vi "Configure Histogram Trigger Source.vi"(8 "error in (no error)":errorcluster {"code" format="%.0x"}, 9 "Histogram Trigger Source (1: Software)":i32(ring)=1 items=["External", "Software", "Immediate", "Pin 1", "Pin 2", "Pin 3"], 10 "Channel Name (1)":string="1", 11 "VISA resource name":refnum<visa-resource-name>) -> (0 "error out":errorcluster {"code" format="%.0x"}, 3 "VISA resource name out":refnum<visa-resource-name>)   [LabVIEW 2010, in "Agilent N6700 Series.lvlib"]
doc: "Configures the trigger source of the histogram function. When the power supply receives a trigger signal on the source you specify, it runs the histogram.\n\n<b>Note:</b>\n\n(1) The VI only applies to models N6781A and N6782A that have the Data Logger function installed.\n\n(2) The histogram function only applies to the N6705B DC Power Analyzer."
uses:
  Agilent N6700 Series.lvlib
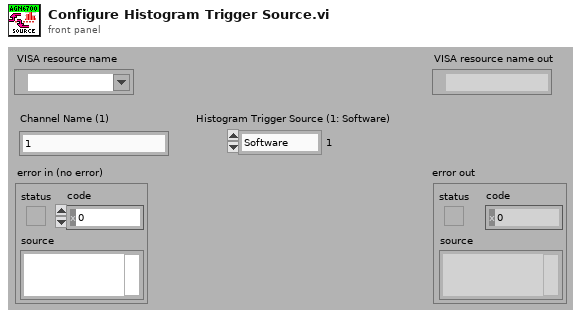
[diagram p1: front panel]
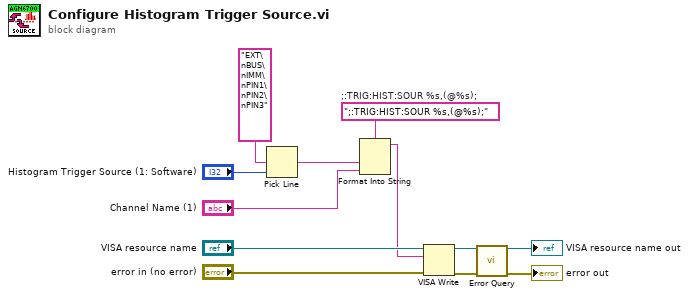
[diagram p0: block diagram]
diagram:
  w12 = ";:TRIG:HIST:SOUR %s,(@%s);"  # ;:TRIG:HIST:SOUR %s,(@%s);
  n1 = Pick Line(multi-line string="EXT\nBUS\nIMM\nPIN1\nPIN2\nPIN3", line index="Histogram Trigger Source (1: Software)") -> (output string=w8:string)  [unwired: 1 in]
  n2 = Format Into String(format string=w12, w8, "Channel Name (1)") -> (resulting string=w6:string)  [unwired: 2 in, 1 out]
  n3 = VISA Write(VISA resource name="VISA resource name", write buffer=w6, error in (no error)="error in (no error)") -> (VISA resource name out=w2:refnum<visa-resource-name>, error out=w1:errorcluster)  [unwired: 1 out]
  n4 = call "Error Query.vi"("VISA resource name"=w2, "error in (no error)"=w1) -> ("VISA resource name out"=→"VISA resource name out":refnum<visa-resource-name>, "error out"=→"error out":errorcluster)  [unwired: 10 in, 2 out]
